vi "Quartic.vi"(4 "ktrap":sgl, 6 "mobX(px/V)":sgl, 10 "alpha quartic":sgl, 11 "Xpx":sgl) -> (3 "counter Force":sgl)   [LabVIEW 2019]
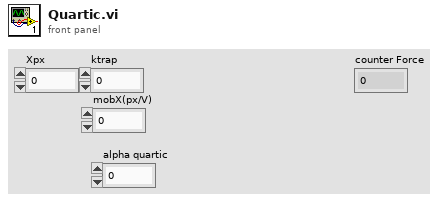
[diagram p1: front panel]
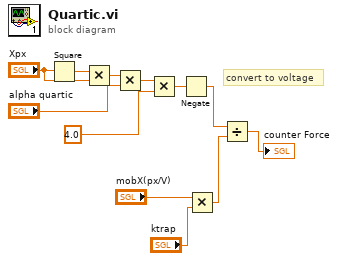
[diagram p0: block diagram]
diagram:
  # "convert to voltage"
  n1 = Square(x="Xpx") -> (x^2=w8:sgl)
  n2 = Multiply(x=w8, y="Xpx") -> (x*y=w6:sgl)
  n3 = Multiply(x=w6, y="alpha quartic") -> (x*y=w4:sgl)
  n4 = Multiply(x=w4, y=sgl 4.0) -> (x*y=w2:sgl)
  n5 = Negate(x=w2) -> (-x=w1:sgl)
  n6 = Multiply(x="mobX(px/V)", y="ktrap") -> (x*y=w10:sgl)
  n7 = Divide(x=w1, y=w10) -> (x/y=→"counter Force":sgl)
